vi "choose standard Test UI.vi"(8 "error in (no error)":errorcluster caption="Fehler (Eingang, kein Fehler)", 10 "TestInterface.lvclass 2":refnum<class "TestInterface.lvclass">, 11 "DeviceInterface Eingang":refnum<class "DeviceInterface.lvclass"> caption="DNL_LabVIEW Object in") -> (0 "error out":errorcluster caption="Fehler (Ausgang)", 2 "TestInterface.lvclass":refnum<class "TestInterface.lvclass">, 3 "DeviceInterface Ausgang":refnum<class "DeviceInterface.lvclass"> caption="DNL_LabVIEW Object out")   [LabVIEW 2013, in "DeviceInterface.lvclass"]
uses:
  DeviceInterface.lvclass
  Tests/TestInterface/TestInterface.lvclass
panel:
  in  "abbrechen":bool
  in  "ok":bool
  in  "Listenfeld":i32(listbox)
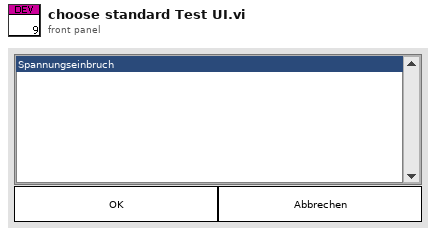
[diagram p1: front panel]
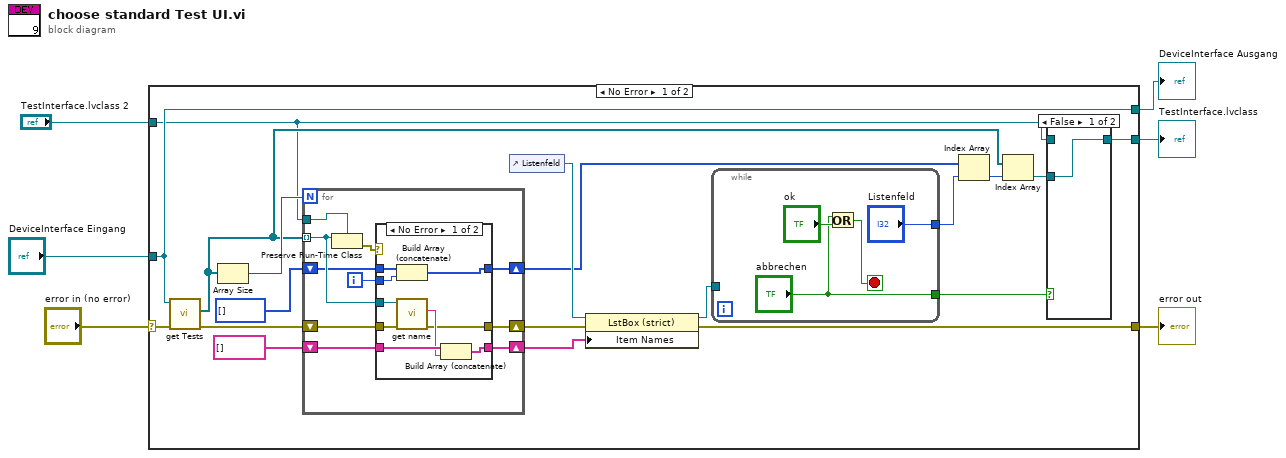
[diagram p0: block diagram]
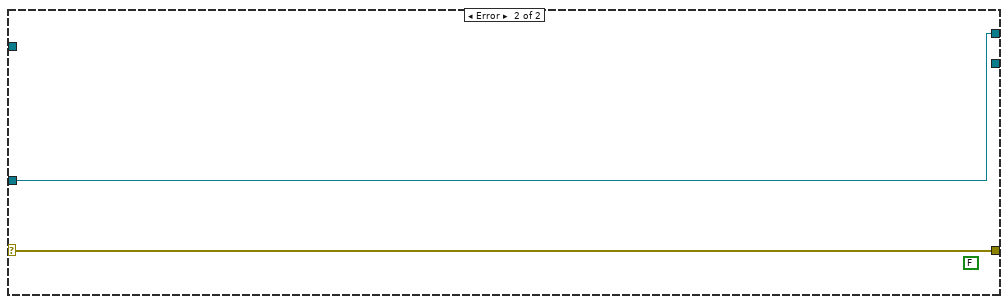
[diagram p4: hidden frame]
diagram:
  n1 = case shown="No Error" "error in (no error)" {
    selector: "error in (no error)" -> [w18 w55]
    tunnel: [w17 w55] -> w5
    tunnel: [w16 w54] -> w3
    tunnel: "DeviceInterface Eingang" -> [w16 w54]
    tunnel: [w12 _] -> w2
    tunnel: "TestInterface.lvclass 2" -> [w11 _]
    frame No Error {
      n2 = call-dynamic "get Tests.vi"("error in (no error)"=w18, "DeviceInterface (Eingang)"=w16) -> ("error out"=w24:errorcluster, "Tests"=w20:refnum<class "TestInterface.lvclass">[])  [unwired: 7 in, 1 out]
      n3 = Array Size(array=w20) -> (size(s)=w25:i32)
      n4 = for {
        N: w25 -> [_]
        tunnel: w20 -> [w37] mode=indexing
        shift-right: [w41] -> w23
        shift-left: string[] [] -> [w40]
        shift-right: [w39] -> w21
        shift-left: w24 -> [w35]
        tunnel: w11 -> [w38]
        shift-right: [w32] -> w10
        shift-left: i32[] [] -> [w33]
        i -> [w34]
        n5 = Preserve Run-Time Class(object in=w37, 2:w38) -> (error out=w36:errorcluster)  [unwired: 1 in, 1 out]
        n6 = case shown="No Error" w36 {
          tunnel: w37 -> [w50 _]
          tunnel: w35 -> [w49 w53]
          tunnel: [w48 w52] -> w41
          tunnel: w40 -> [w47 w52]
          tunnel: [w45 w53] -> w39
          tunnel: w34 -> [w44 _]
          tunnel: w33 -> [w43 w51]
          tunnel: [w42 w51] -> w32
          frame No Error {
            n7 = Build Array (concatenate)(w43, w44) -> (w42:i32[])
            n8 = call-dynamic "get name.vi"("error in (no error)"=w49, "TestInterface (Eingang)"=w50) -> ("error out"=w45:errorcluster, "name"=w46:string)  [unwired: 7 in, 1 out]
            n9 = Build Array (concatenate)(w47, w46) -> (w48:string[])
          }
          frame Error {
          }
        }
      }
      n10 = control-ref of="Listenfeld"() -> (w22:refnum<vi>)
      n11 = property class="LstBox (strict)"(reference=w22, error in=w21, "Item Names"=w23) -> (reference out=w19:refnum<vi>, error out=w17:errorcluster)
      n12 = while {
        tunnel: ["Listenfeld"] -> w9
        tunnel: w19 -> [_]
        tunnel: ["abbrechen"] -> w14
        stop <- w29 stop-if-true
        n13 = Or(x="abbrechen", y="ok") -> (x .or. y?=w29:bool)
      }
      n14 = Index Array(array=w10, index=w9) -> (element=w8:i32)
      n15 = Index Array(array=w20, index=w8) -> (element=w13:refnum<class "TestInterface.lvclass">)
      n16 = case shown="False" w14 {
        tunnel: w13 -> [w26 _]
        tunnel: [w26 w27] -> w12
        tunnel: w11 -> [_ w27]
        frame False {
        }
        frame True {
        }
      }
    }
    frame Error {
      (unwired) FALSE ("abbrechen")
    }
  }
  "error out" <- w5
  "DeviceInterface Ausgang" <- w3
  "TestInterface.lvclass" <- w2
